vi "compute_parameters.vi"(10 "Target Pulse Duration (ms)":dbl, 11 "Target Peak Displacement (mm)":dbl) -> (1 "Acceleration (decimicrons/s2)":dbl, 2 "Velocity (decimicrons/s)":dbl, 3 "Position at Peak (decimicrons)":dbl)   [LabVIEW 2014]
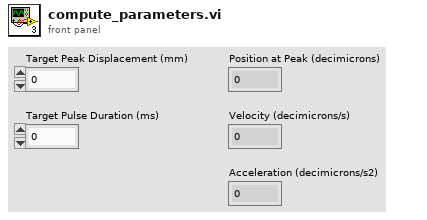
[diagram p1: front panel]
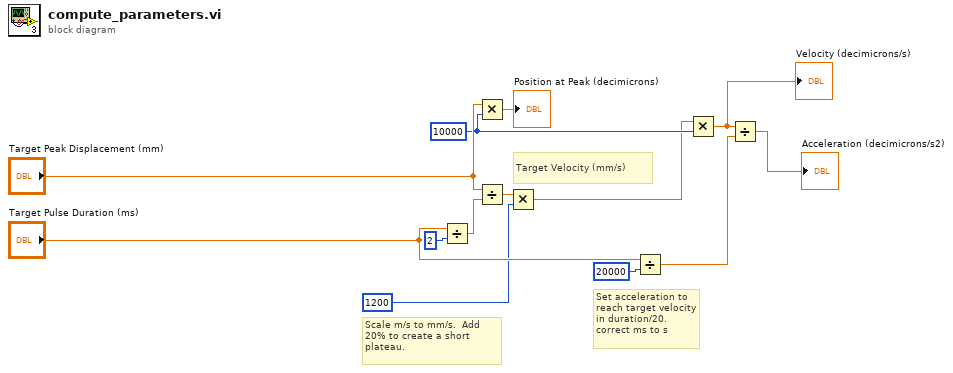
[diagram p0: block diagram]
diagram:
  w6 = 10000
  # "Scale m/s to mm/s.  Add 20% to create a short plateau."
  # "Target Velocity (mm/s)"
  # "Set acceleration to reach target velocity in duration/20.  correct ms to s"
  n1 = Divide(x="Target Pulse Duration (ms)", y=2) -> (x/y=w2:dbl)
  n2 = Multiply(x="Target Peak Displacement (mm)", y=w6) -> (x*y=→"Position at Peak (decimicrons)":dbl)
  n3 = Divide(x="Target Peak Displacement (mm)", y=w2) -> (x/y=w3:dbl)
  n4 = Multiply(x=w3, y=1200) -> (x*y=w4:dbl)
  n5 = Divide(x="Target Pulse Duration (ms)", y=20000) -> (x/y=w11:dbl)
  n6 = Multiply(x=w4, y=w6) -> (x*y=w12:dbl)
  "Velocity (decimicrons/s)" <- w12
  n7 = Divide(x=w12, y=w11) -> (x/y=→"Acceleration (decimicrons/s2)":dbl)
